vi "test.vi"() -> ()   [LabVIEW 2022 SP3, in "SingleStepTestV2.lvlib" / "SingleStepTestV2.lvclass"]
uses:
  SingleStepTestV2.lvclass
panel:
  in  "单步调试":T8={"注射泵"=enum."注入", "阀口选择"=enum."V1", "灯"=enum."未选择", "ADC值"=enum."未选择", "数值"=4000, "项目输入"=0, "控温"=enum."未选择", "外设选择"=enum."未选择", "外设选择2"={"V9-1"=FALSE, "V9-2"=FALSE}} {"项目输入" items=["氨氮"=131]}
  out "数组":u16[](array[numeric]) format="%04x"
  in  "布尔":bool
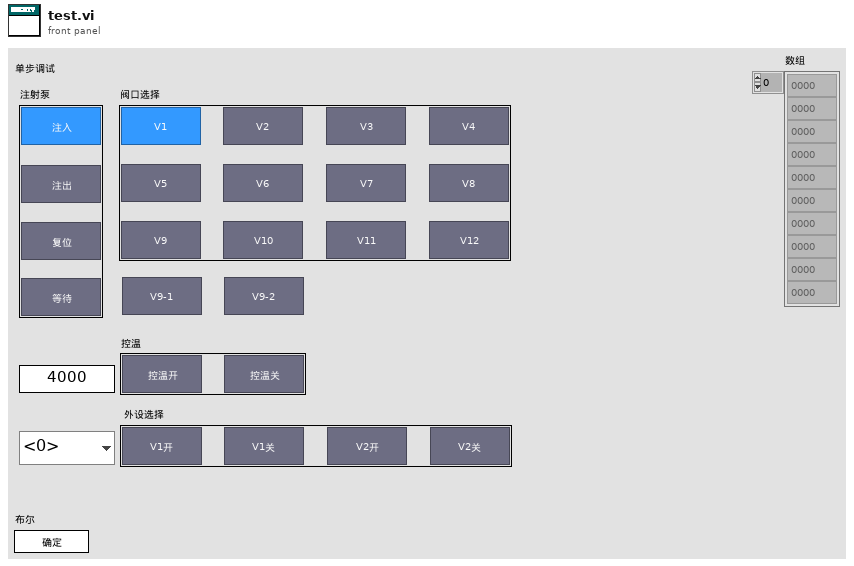
[diagram p1: front panel]
types:
  T1 = typedef "SingleStepTestV2.lvlib/SingleStepTestV2.lvclass/注射泵操作.ctl" = enum32{"复位", "注入", "注出", "等待"}
  T2 = typedef "SingleStepTestV2.lvlib/SingleStepTestV2.lvclass/阀口操作.ctl" = enum32{"未选择", "V1", "V2", "V3", "V4", "V5", "V6", "V7", "V8", "V9", "V10", "V11", "V12"}
  T3 = typedef "SingleStepTestV2.lvlib/SingleStepTestV2.lvclass/灯选择.ctl" = enum32{"未选择", "520", "660", "加热恒温", "氙灯/紫灯"}
  T4 = typedef "SingleStepTestV2.lvlib/SingleStepTestV2.lvclass/ADC选择.ctl" = enum32{"未选择", "ADC0", "降温温度", "消解温度", "光谱/ADC1"}
  T5 = typedef "SingleStepTestV2.lvlib/SingleStepTestV2.lvclass/控温操作.ctl" = enum32{"未选择", "控温开", "控温关"}
  T6 = typedef "SingleStepTestV2.lvlib/SingleStepTestV2.lvclass/外设选择.ctl" = enum32{"未选择", "V1开", "V1关", "V2开", "V2关"}
  T7 = typedef "SingleStepTestV2.lvlib/SingleStepTestV2.lvclass/外设选择2.ctl" = cluster{"V9-1":bool, "V9-2":bool}
  T8 = cluster{"注射泵":T1, "阀口选择":T2, "灯":T3, "ADC值":T4, "数值":i16, "项目输入":u16, "控温":T5, "外设选择":T6, "外设选择2":T7}
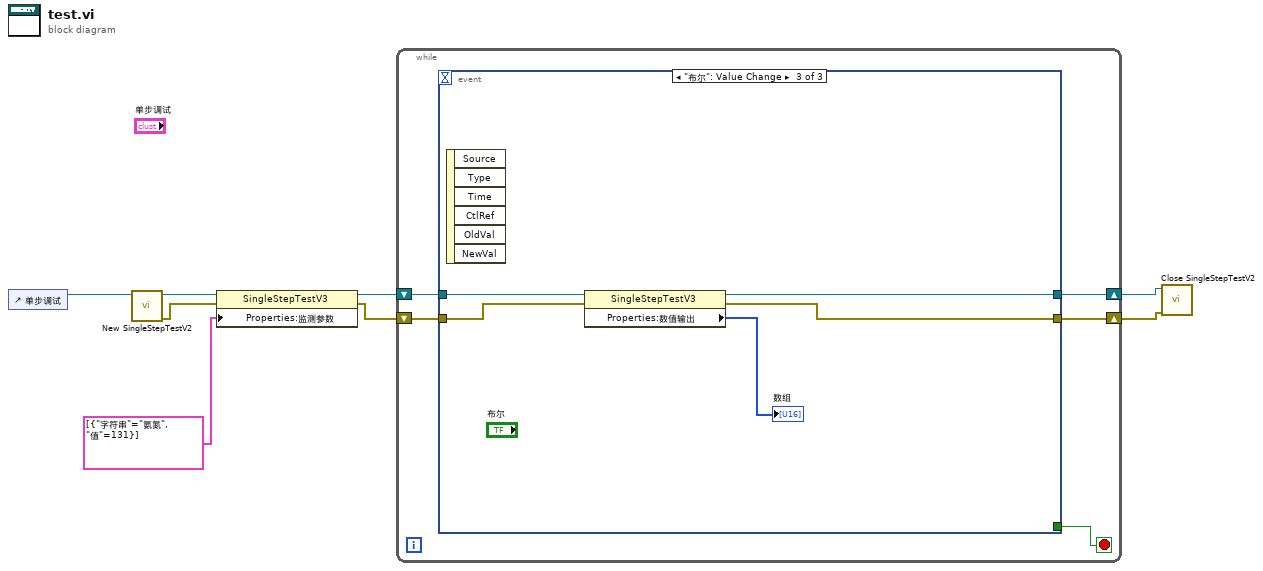
[diagram p0: block diagram]
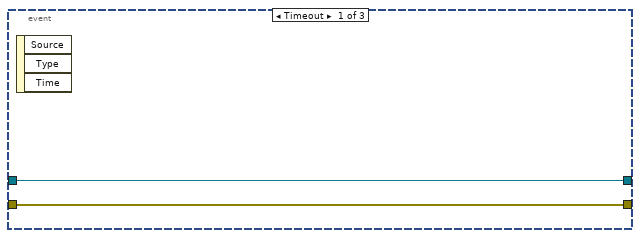
[diagram p2: hidden frame]
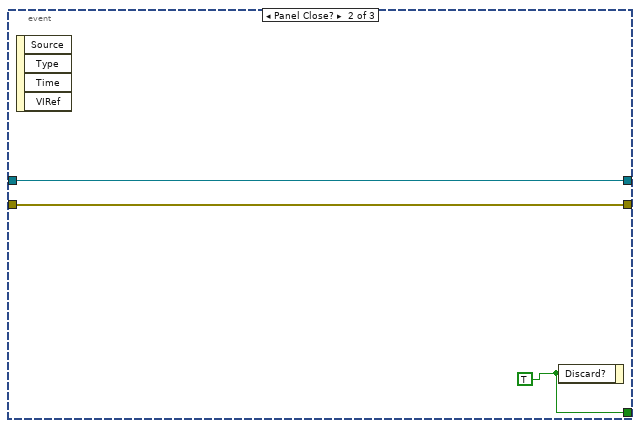
[diagram p3: hidden frame]
diagram:
  n1 = control-ref of="单步调试"() -> (w3:refnum<vi>)
  n2 = call "New SingleStepTestV2.vi"("Reference"=w3) -> ("error out"=w4:errorcluster, "SingleStepTestV3 out"=w2:refnum<class "SingleStepTestV2.lvclass">)  [unwired: 9 in]
  n3 = property class="SingleStepTestV3"(reference=w2, error in=w4, "Properties:监测参数"=cluster{"字符串":string, "值":u16}[] [{"字符串"="氨氮", "值"=131}] ("字符串与值")) -> (reference out=w6:refnum<class "SingleStepTestV2.lvclass">, error out=w5:errorcluster)
  n4 = while {
    shift-right: [w10] -> w8
    shift-left: w6 -> [w13]
    shift-right: [w9] -> w7
    shift-left: w5 -> [w12]
    stop <- w11 stop-if-true
    n5 = event shown="[2] \"布尔\": Value Change" {
      selector: _ -> [_ _ _]
      dyn-events: _ -> [_ _ _]
      timeout: _ -> [_ _ _]
      tunnel: w13 -> [w15 w17 w23]
      tunnel: w12 -> [w14 w16 w22]
      tunnel: [_ w18 _] -> w11
      tunnel: [w15 w17 w20] -> w10
      tunnel: [w14 w16 w21] -> w9
      event Timeout {
        n6 = event-data() -> ()  [unwired: 1 in, 3 out]
      }
      event Panel Close? {
        w18 = TRUE
        n7 = event-data() -> ()  [unwired: 1 in, 4 out]
        n8 = event-data("Discard?"=w18) -> ()  [unwired: 1 in, 1 out]
      }
      event "布尔": Value Change {
        n9 = event-data() -> ()  [unwired: 1 in, 6 out]
        n10 = property class="SingleStepTestV3"(reference=w23, error in=w22) -> (reference out=w20:refnum<class "SingleStepTestV2.lvclass">, error out=w21:errorcluster, "Properties:数值输出"=→"数组":u16[])
      }
    }
  }
  n11 = call "Close SingleStepTestV2.vi"("error in (no error)"=w7, "SingleStepTestV3 in"=w8) -> ()  [unwired: 9 in, 1 out]
